vi "INIT 1.1.vi"(8 "error in (no error)":errorcluster, 11 "VISA resource name":refnum<visa-resource-name>) -> (0 "error out":errorcluster, 3 "VISA resource name out":refnum<visa-resource-name>)   [LabVIEW 2014, in "CAP-USB.lvlib"]
doc: "Envia el codigo de inicializacion del CAP-USB 1.0 en hexadecimal"
uses:
  CAP-USB.lvlib
panel:
  in  "Codigo de inicializacion":string="W\u0003\u0003W\u0003\u0001\u0000W\u0003\u0002\u0000W\u0003\u0007W\u0003\u0005\u0000W\u0003\u0006\u0000W\u0003\u000bW\u0003\t\u0000W\u0003\n\u0000W\u0003\u000fW\u0003\r\u0000W\u0003\u000e\u0000W\u0003\u000bW\u0003\n\u0001W\u0003\u0013W\u0003\u0012ðW\u0003\u0017W\u0003\u0014ÿW\u0003\u0015\u0000s"
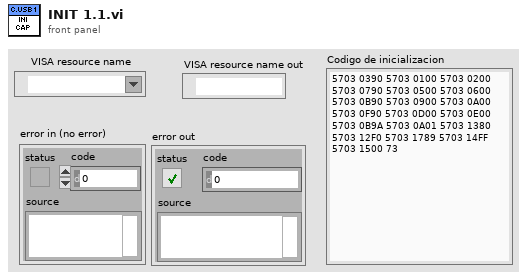
[diagram p1: front panel]
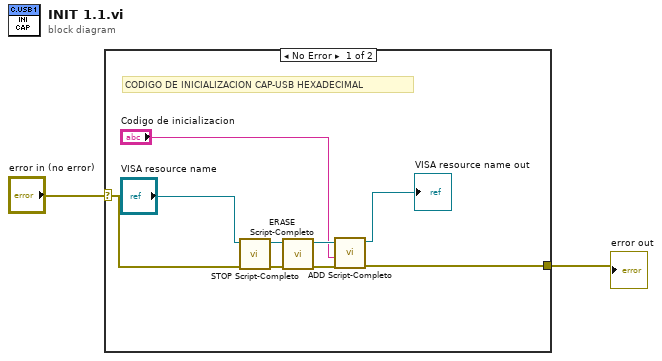
[diagram p0: block diagram]
diagram:
  n1 = case shown="No Error" "error in (no error)" {
    selector: "error in (no error)" -> [w3 w12]
    tunnel: [w4 w12] -> w2
    frame No Error {
      # "CODIGO DE INICIALIZACION CAP-USB HEXADECIMAL"
      n2 = call "STOP Script-Completo.vi"("error in (no error)"=w3, "VISA resource name"="VISA resource name") -> ("error out"=w9:errorcluster, "VISA resource name out"=w10:refnum<visa-resource-name>)  [unwired: 8 in]
      n3 = call "ERASE Script-Completo.vi"("error in (no error)"=w9, "VISA resource name"=w10) -> ("error out"=w8:errorcluster, "VISA resource name out"=w7:refnum<visa-resource-name>)  [unwired: 8 in]
      n4 = call "ADD Script-Completo.vi"("error in (no error)"=w8, "Datos a agregar"="Codigo de inicializacion", "VISA resource name"=w7) -> ("error out"=w4:errorcluster, "VISA resource name out"=→"VISA resource name out":refnum<visa-resource-name>)  [unwired: 7 in]
    }
    frame Error {
    }
  }
  "error out" <- w2
